vi "Set Measurement.vi"(6 "Escala":dbl, 8 "error in (no error)":errorcluster, 9 "Range ON/OFF":bool, 10 "Grandeza Elétrica":string, 11 "8846A in":refnum<class "8846A.lvclass">) -> (0 "error out":errorcluster, 3 "8846A out":refnum<class "8846A.lvclass">)   [LabVIEW 2015, in "8846A.lvclass"]
uses:
  8846A.lvclass
  <instrlib>/Fluke 884X Series/Fluke 884X Series.lvlib
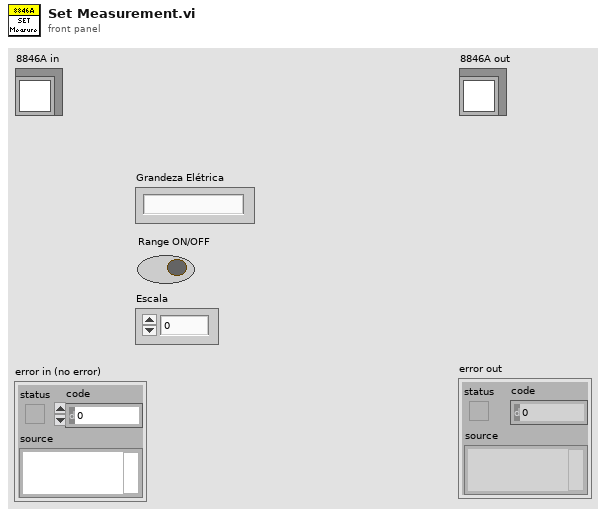
[diagram p1: front panel]
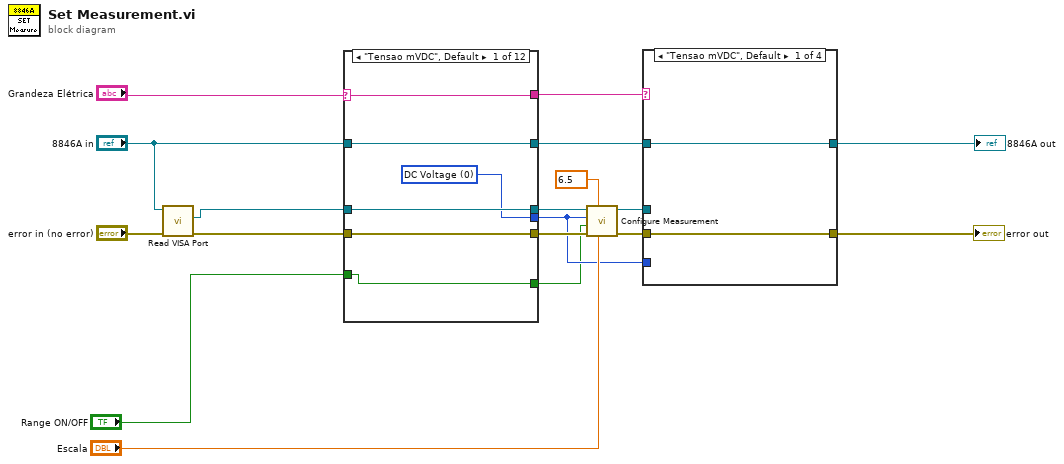
[diagram p0: block diagram]
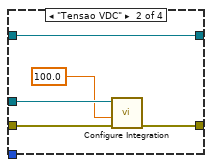
[diagram p2: hidden frame]
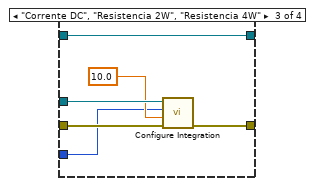
[diagram p3: hidden frame]
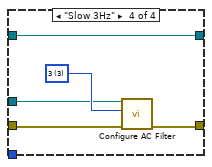
[diagram p4: hidden frame]
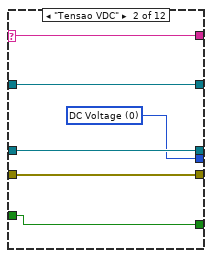
[diagram p5: hidden frame]
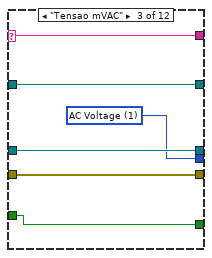
[diagram p6: hidden frame]
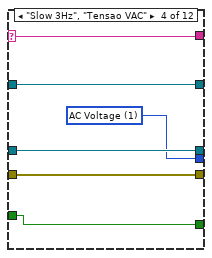
[diagram p7: hidden frame]
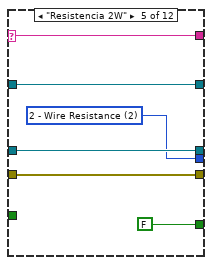
[diagram p8: hidden frame]
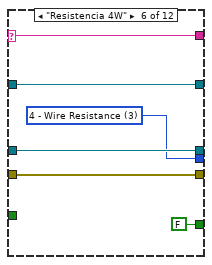
[diagram p9: hidden frame]
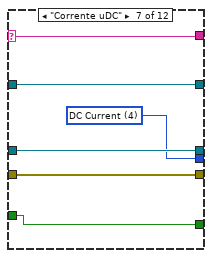
[diagram p10: hidden frame]
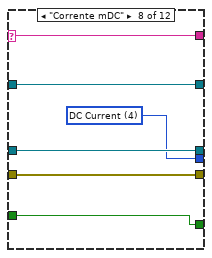
[diagram p11: hidden frame]
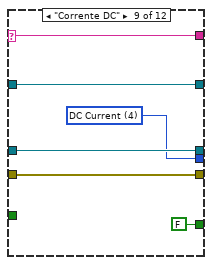
[diagram p12: hidden frame]
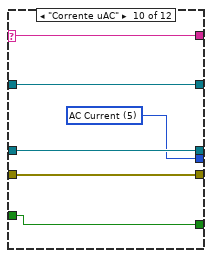
[diagram p13: hidden frame]
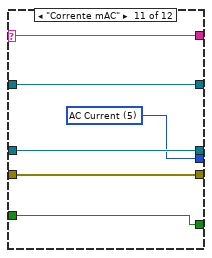
[diagram p14: hidden frame]
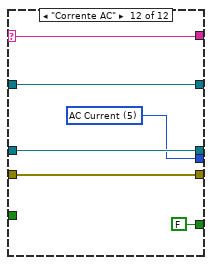
[diagram p15: hidden frame]
diagram:
  w7 = 6.5 items=["4.5"=4.5, "5.5"=5.5, "6.5"=6.5] ("Manual Resolution (5.5 Digits)")
  n1 = call-dynamic "Read VISA Port.vi"("error in (no error)"="error in (no error)", "Device in"="8846A in") -> ("error out"=w12:errorcluster, "VISA Port"=w11:refnum<visa-resource-name>)  [unwired: 7 in, 1 out]
  n2 = case shown="\"Tensao mVDC\", Default" "Grandeza Elétrica" {
    selector: "Grandeza Elétrica" -> [w20 w26 w32 w38 w44 w50 w56 w62 w68 w74 w80 w86]
    tunnel: w12 -> [w23 w29 w35 w41 w47 w53 w59 w65 w71 w77 w83 w89]
    tunnel: w11 -> [w24 w30 w36 w42 w48 w54 w60 w66 w72 w78 w84 w90]
    tunnel: [w24 w30 w36 w42 w48 w54 w60 w66 w72 w78 w84 w90] -> w9
    tunnel: [w23 w29 w35 w41 w47 w53 w59 w65 w71 w77 w83 w89] -> w8
    tunnel: "8846A in" -> [w22 w28 w34 w40 w46 w52 w58 w64 w70 w76 w82 w88]
    tunnel: [w22 w28 w34 w40 w46 w52 w58 w64 w70 w76 w82 w88] -> w5
    tunnel: [w21 w27 w33 w39 w45 w51 w57 w63 w69 w75 w81 w87] -> w2
    tunnel: [w20 w26 w32 w38 w44 w50 w56 w62 w68 w74 w80 w86] -> w6
    tunnel: [w19 w25 w31 w37 FALSE FALSE ("Range ON/OFF") w55 w61 FALSE ("Range ON/OFF") w73 w79 FALSE ("Range ON/OFF")] -> w1
    tunnel: "Range ON/OFF" -> [w19 w25 w31 w37 _ _ w55 w61 _ w73 w79 _]
    frame "Tensao mVDC", Default {
      w21 = u16 0 items=["DC Voltage", "AC Voltage", "2 - Wire Resistance", "4 - Wire Resistance", "DC Current", "AC Current", "Frequency", "Period", "Continuity", "Diode Checking", "VDC:VDC Ratio", "Temperature", "Capacitance"] ("Function (0: DC Voltage)")
    }
    frame "Tensao VDC" {
      w27 = u16 0 items=["DC Voltage", "AC Voltage", "2 - Wire Resistance", "4 - Wire Resistance", "DC Current", "AC Current", "Frequency", "Period", "Continuity", "Diode Checking", "VDC:VDC Ratio", "Temperature", "Capacitance"] ("Function (0: DC Voltage)")
    }
    frame "Tensao mVAC" {
      w33 = u16 1 items=["DC Voltage", "AC Voltage", "2 - Wire Resistance", "4 - Wire Resistance", "DC Current", "AC Current", "Frequency", "Period", "Continuity", "Diode Checking", "VDC:VDC Ratio", "Temperature", "Capacitance"] ("Function (0: DC Voltage)")
    }
    frame "Slow 3Hz", "Tensao VAC" {
      w39 = u16 1 items=["DC Voltage", "AC Voltage", "2 - Wire Resistance", "4 - Wire Resistance", "DC Current", "AC Current", "Frequency", "Period", "Continuity", "Diode Checking", "VDC:VDC Ratio", "Temperature", "Capacitance"] ("Function (0: DC Voltage)")
    }
    frame "Resistencia 2W" {
      w45 = u16 2 items=["DC Voltage", "AC Voltage", "2 - Wire Resistance", "4 - Wire Resistance", "DC Current", "AC Current", "Frequency", "Period", "Continuity", "Diode Checking", "VDC:VDC Ratio", "Temperature", "Capacitance"] ("Function (0: DC Voltage)")
    }
    frame "Resistencia 4W" {
      w51 = u16 3 items=["DC Voltage", "AC Voltage", "2 - Wire Resistance", "4 - Wire Resistance", "DC Current", "AC Current", "Frequency", "Period", "Continuity", "Diode Checking", "VDC:VDC Ratio", "Temperature", "Capacitance"] ("Function (0: DC Voltage)")
    }
    frame "Corrente uDC" {
      w57 = u16 4 items=["DC Voltage", "AC Voltage", "2 - Wire Resistance", "4 - Wire Resistance", "DC Current", "AC Current", "Frequency", "Period", "Continuity", "Diode Checking", "VDC:VDC Ratio", "Temperature", "Capacitance"] ("Function (0: DC Voltage)")
    }
    frame "Corrente mDC" {
      w63 = u16 4 items=["DC Voltage", "AC Voltage", "2 - Wire Resistance", "4 - Wire Resistance", "DC Current", "AC Current", "Frequency", "Period", "Continuity", "Diode Checking", "VDC:VDC Ratio", "Temperature", "Capacitance"] ("Function (0: DC Voltage)")
    }
    frame "Corrente DC" {
      w69 = u16 4 items=["DC Voltage", "AC Voltage", "2 - Wire Resistance", "4 - Wire Resistance", "DC Current", "AC Current", "Frequency", "Period", "Continuity", "Diode Checking", "VDC:VDC Ratio", "Temperature", "Capacitance"] ("Function (0: DC Voltage)")
    }
    frame "Corrente uAC" {
      w75 = u16 5 items=["DC Voltage", "AC Voltage", "2 - Wire Resistance", "4 - Wire Resistance", "DC Current", "AC Current", "Frequency", "Period", "Continuity", "Diode Checking", "VDC:VDC Ratio", "Temperature", "Capacitance"] ("Function (0: DC Voltage)")
    }
    frame "Corrente mAC" {
      w81 = u16 5 items=["DC Voltage", "AC Voltage", "2 - Wire Resistance", "4 - Wire Resistance", "DC Current", "AC Current", "Frequency", "Period", "Continuity", "Diode Checking", "VDC:VDC Ratio", "Temperature", "Capacitance"] ("Function (0: DC Voltage)")
    }
    frame "Corrente AC" {
      w87 = u16 5 items=["DC Voltage", "AC Voltage", "2 - Wire Resistance", "4 - Wire Resistance", "DC Current", "AC Current", "Frequency", "Period", "Continuity", "Diode Checking", "VDC:VDC Ratio", "Temperature", "Capacitance"] ("Function (0: DC Voltage)")
    }
  }
  n3 = call <instrlib>:"Configure Measurement.vi"("Manual Range (1.0)"="Escala", "Manual Resolution (5.5 Digits)"=w7, "error in (no error)"=w8, "Auto Range (T:Enable)"=w1, "Function (0: DC Voltage)"=w2, "VISA resource name"=w9) -> ("error out"=w3:errorcluster, "VISA resource name out"=w4:refnum<visa-resource-name>)  [unwired: 4 in]
  n4 = case shown="\"Tensao mVDC\", Default" w6 {
    tunnel: w5 -> [w92 w97 w103 w108]
    tunnel: [w92 w97 w103 w108] -> w13
    tunnel: w4 -> [_ w96 w102 w106]
    tunnel: w3 -> [w91 w94 w100 w105]
    tunnel: [w91 w93 w99 w104] -> w14
    tunnel: w2 -> [_ _ w98 _]
    frame "Tensao mVDC", Default {
    }
    frame "Tensao VDC" {
      w95 = 100.0 items=["0.001"=0.001, "0.002"=0.002, "0.006"=0.006, "0.02"=0.02, "0.06"=0.06, "0.2"=0.2, "1"=1.0, "10"=10.0, "100"=100.0] ("Integration Time (1 PLCs)")
      n5 = call <instrlib>:"Configure Integration.vi"("error in (no error)"=w94, "Integration Time (10 PLCs)"=w95, "VISA resource name"=w96) -> ("error out"=w93:errorcluster)  [unwired: 7 in, 1 out]
    }
    frame "Corrente DC", "Resistencia 2W", "Resistencia 4W" {
      w101 = 10.0 items=["0.001"=0.001, "0.002"=0.002, "0.006"=0.006, "0.02"=0.02, "0.06"=0.06, "0.2"=0.2, "1"=1.0, "10"=10.0, "100"=100.0] ("Integration Time (1 PLCs)")
      n6 = call <instrlib>:"Configure Integration.vi"("error in (no error)"=w100, "Integration Time (10 PLCs)"=w101, "Function (0: DC Voltage)"=w98, "VISA resource name"=w102) -> ("error out"=w99:errorcluster)  [unwired: 6 in, 1 out]
    }
    frame "Slow 3Hz" {
      w107 = 3 items=["3"=3, "20"=20, "200"=200] ("AC Filter Bandwidth (20 Hz)")
      n7 = call <instrlib>:"Configure AC Filter.vi"("error in (no error)"=w105, "AC Filter Bandwidth (20 Hz)"=w107, "VISA resource name"=w106) -> ("error out"=w104:errorcluster)  [unwired: 7 in, 1 out]
    }
  }
  "error out" <- w14
  "8846A out" <- w13
